vi "DEBUG Query VI.vi"() -> ()   [LabVIEW 2013]
uses:
  <vilib>/Utility/traverseref.llb/VI Scripting - Traverse.lvlib
  <vilib>/Utility/traverseref.llb/TRef TravTarget.ctl
panel:
  out "Names":string[](array[string])
  out "IDs":u32[](array[numeric])
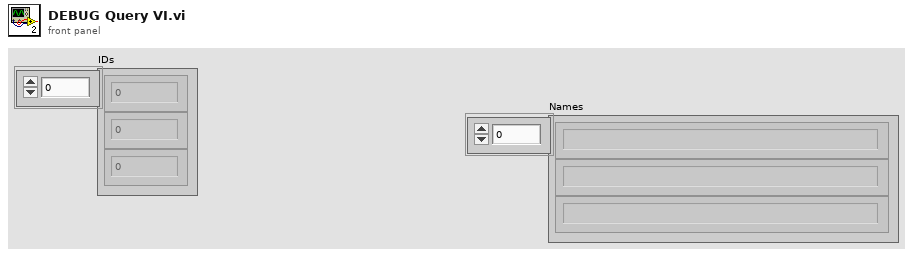
[diagram p1: front panel]
types:
  T1 = typedef "TRef TravTarget.ctl" = enum16{"FP", "BD", "Other"}
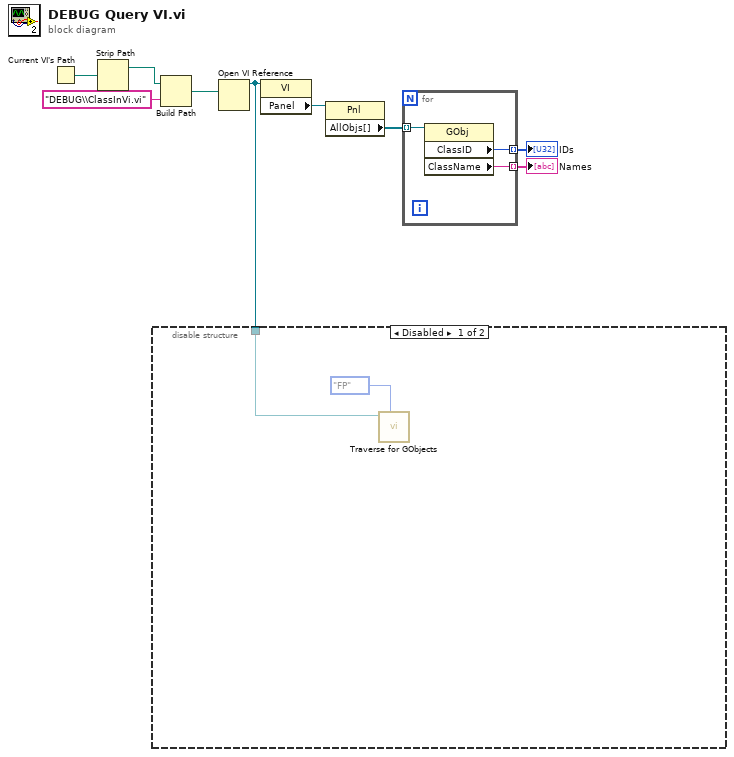
[diagram p0: block diagram]
diagram:
  n1 = Current VI's Path() -> (path=w9:path)
  n2 = Strip Path(path=w9) -> (stripped path=w8:path)  [unwired: 1 out]
  n3 = Build Path(base path=w8, name or relative path="DEBUG\\ClassInVi.vi") -> (appended path=w6:path)
  n4 = Open VI Reference(vi path=w6) -> (vi reference=w1:refnum<vi>)  [unwired: 5 in, 1 out]
  n5 = disable-structure shown="Disabled" {
    disable-tunnel: w1 -> [w11 _]
    frame Disabled {
      n6 = call <vilib>:"Traverse for GObjects.vi"("Traverse Target"=TRef_TravTarget."FP", "VI Refnum"=w11) -> ()  [unwired: 6 in, 4 out]
    }
    frame Enabled {
    }
  }
  n7 = property class="VI"(reference=w1) -> ("Panel"=w5:refnum<vi>)  [unwired: 1 in, 2 out]
  n8 = property class="Pnl"(reference=w5) -> ("AllObjs[]"=w4:refnum<vi>[])  [unwired: 1 in, 2 out]
  n9 = for {
    tunnel: w4 -> [w14] mode=indexing
    tunnel: [w13] -> w3 mode=indexing
    tunnel: [w12] -> w2 mode=indexing
    n10 = property class="GObj"(reference=w14) -> ("ClassID"=w13:u32, "ClassName"=w12:string)  [unwired: 1 in, 2 out]
  }
  "IDs" <- w3
  "Names" <- w2
